vi "test-Signal With Safe Period.vi"() -> ()   [LabVIEW 2017]
uses:
  caadbb02-b5a9-4500-a158-ff12e9729595.vi
  Signal/Turn F Immediatly But Ture T with Latency.vi/5093cefc-d3d2-4eb3-bc00-370220dfee7f.vi
  Signal/Turn F Immediatly But Ture T with Latency.vi/d8dc2e1a-5964-4f74-9887-ef2f57e1a81f.vi
  Signal/Turn T Immediatly But Ture F with Latency.vi/5093cefc-d3d2-4eb3-bc00-370220dfee7f.vi
  Signal/Turn T Immediatly But Ture F with Latency.vi/be714cb1-a87c-4b18-bbea-1129bb0f91bd.vi
  caadbb02-b5a9-4500-a158-ff12e9729595.vi/b4d18e63-bf87-453f-a2fc-a60400babe92.vi
  caadbb02-b5a9-4500-a158-ff12e9729595.vi/aa9064e7-7b56-4afb-ab33-c56135921fd1.vi
panel:
  out "signal(safe) 3":bool
  out "Turn T Immediatly But Ture F with Latency.vi":bool
  out "Turn F Immediatly But Ture T with Latency.vi":bool
  out "变化过去时间(ms) 1":u32
  out "变化过去时间(ms) 3":u32
  out "变化过去时间(ms) 2":u32
  in  "reset":bool
  in  "Signal":bool
  in  "stop":bool
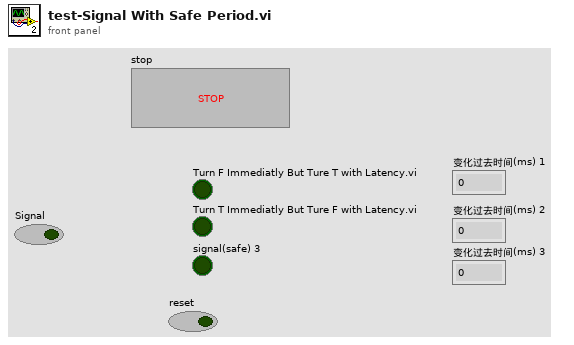
[diagram p1: front panel]
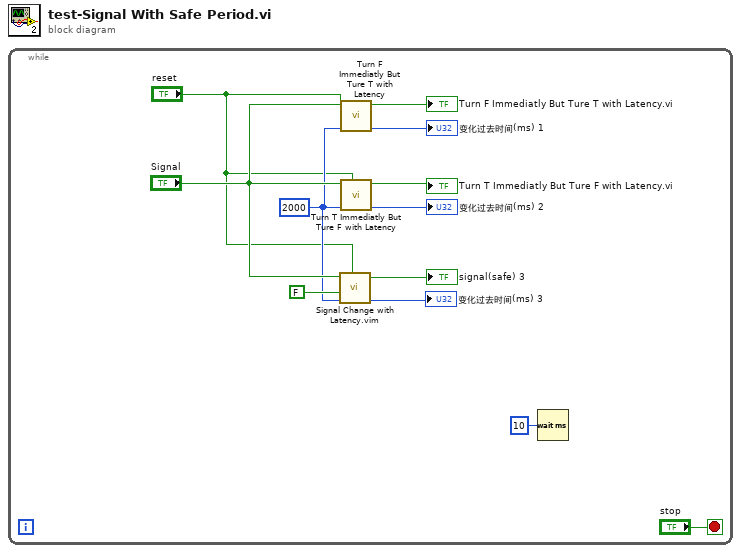
[diagram p0: block diagram]
diagram:
  n1 = while {
    stop <- "stop" stop-if-true
    w3 = u32 2000 ("计时时长(ms)")
    n2 = call "Signal Change with Latency.vim"("reset(F)"="reset", "计时时长(ms)"=w3, "reset value"=FALSE, "Signal"="Signal") -> ("变化过去时间(ms)"=→"变化过去时间(ms) 3":u32, "signal(safe)"=→"signal(safe) 3":bool)  [unwired: 6 in]
    n3 = call "Turn F Immediatly But Ture T with Latency.vi"("Reset(F)"="reset", "计时时长(ms)"=w3, "Signal"="Signal") -> ("变化过去时间(ms)"=→"变化过去时间(ms) 1":u32, "signal(safe)"=→"Turn F Immediatly But Ture T with Latency.vi":bool)  [unwired: 7 in]
    n4 = call "Turn T Immediatly But Ture F with Latency.vi"("Reset(F)"="reset", "计时时长(ms)"=w3, "Signal"="Signal") -> ("变化过去时间(ms)"=→"变化过去时间(ms) 2":u32, "signal(safe)"=→"Turn T Immediatly But Ture F with Latency.vi":bool)  [unwired: 7 in]
    n5 = Wait (ms)(milliseconds to wait=u32 10) -> ()  [unwired: 1 out]
  }
